vi "Stage Reference Follower.vi"(6 "stop":bool, 8 "Stage PID Cluster":T1={"Stage Z PID"={"Kp"=0.0005, "Kd"=0.001, "Ki"=0.0}, "Stage Y PID"={"Kp"=0.0003, "Kd"=0.01, "Ki"=0.0}, "Stage X PID"={"Kp"=0.0003, "Kd"=0.01, "Ki"=0.0}}, 9 "Stage cmd Posit [mm]":dbl[](array[numeric])=[6.0, 6.0, 6.0], 10 "error in":errorcluster, 11 "FPGA VI Reference In":refnum<k20>) -> (1 "Stage out Posit [mm]":dbl[](array[numeric])=[12.0, 0.0, 0.0], 2 "error out":errorcluster, 3 "FPGA VI Reference Out":refnum<k20>)   [LabVIEW 2016]
uses:
  <vilib>/Utility/error.llb/Error Cluster From Error Code.vi
  <vilib>/rvi/errors/niLvFpgaAdjustHostInterfaceError.vi
  <vilib>/rvi/interface/nirviReadWriteControl/nirviReadWriteControl.xnode
  FPGA Bitfiles/IRISSTrack_FPGATarget2_IRISSFPGAIORIO_4NTO9ubhv-c.lvbitx
  IRISS_FPGA_IO_RIO.vi
  Library/jmslib.lvlib
  NiFpgaLv.dll
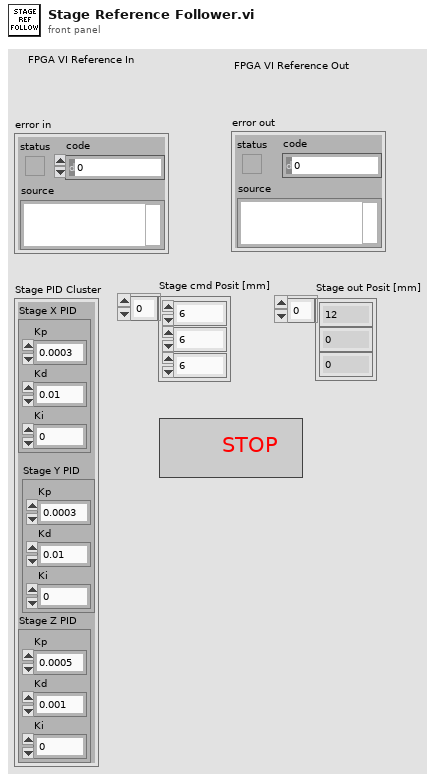
[diagram p1: front panel]
types:
  T1 = cluster{"Stage Z PID":cluster{"Kp":dbl, "Kd":dbl, "Ki":dbl}, "Stage Y PID":cluster{"Kp":dbl, "Kd":dbl, "Ki":dbl}, "Stage X PID":cluster{"Kp":dbl, "Kd":dbl, "Ki":dbl}}
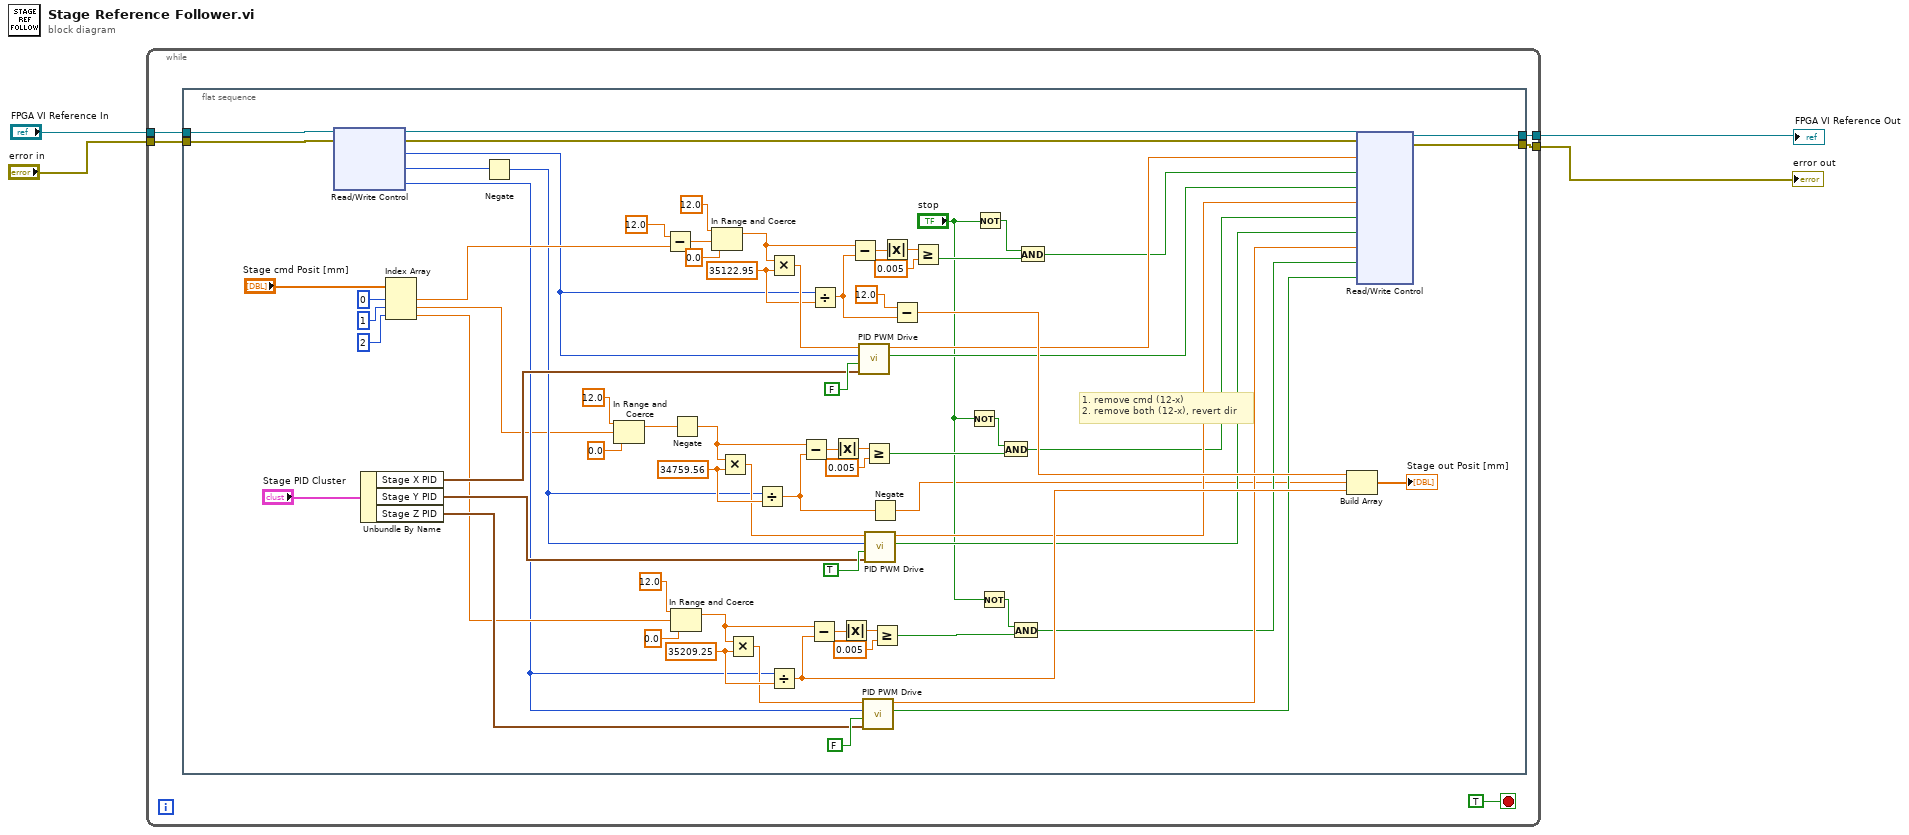
[diagram p0: block diagram]
diagram:
  n1 = while {
    tunnel: "FPGA VI Reference In" -> [w9]
    tunnel: "error in" -> [w8]
    tunnel: [w7] -> w1
    tunnel: [w6] -> w4
    stop <- TRUE stop-if-true
    n2 = flat-sequence {
      tunnel: w9 -> [w83]
      tunnel: w8 -> [w82]
      tunnel: [w22] -> w7
      tunnel: [w21] -> w6
      frame #0 {
        w49 = 35209.25 ("y")
        w63 = 34759.56 ("y")
        w78 = 35122.95 ("y")
        # "1. remove cmd (12-x)\n2. remove both (12-x), revert dir"
        n3 = xnode "Read/Write Control"("FPGA VI Reference In"=w83, "error in"=w82) -> ("FPGA VI Reference Out"=w24:refnum<k20>, "error out"=w23:errorcluster, "Position X"=w31:i32, "Position Y"=w16:i32, "Position Z"=w20:i32)
        n4 = Unbundle By Name("Stage PID Cluster") -> ("Stage X PID"=w56:cluster{"Kp":dbl, "Kd":dbl, "Ki":dbl}, "Stage Y PID"=w55:cluster{"Kp":dbl, "Kd":dbl, "Ki":dbl}, "Stage Z PID"=w43:cluster{"Kp":dbl, "Kd":dbl, "Ki":dbl})
        n5 = Index Array(array="Stage cmd Posit [mm]", index #1=0 ("index"), index #2=1 ("index"), index #3=2 ("index")) -> (element #1=w68:dbl, element #2=w10:dbl, element #3=w39:dbl)
        n6 = Negate(x=w16) -> (-x=w15:i32)
        n7 = In Range and Coerce(upper limit=12.0, x=w10, lower limit=0.0) -> (coerced(x)=w12:dbl)  [unwired: 1 out]
        n8 = Subtract(x=12.0 ("upper limit"), y=w68) -> (x-y=w72:dbl)
        n9 = In Range and Coerce(upper limit=12.0, x=w39, lower limit=0.0) -> (coerced(x)=w51:dbl)  [unwired: 1 out]
        n10 = Negate(x=w12) -> (-x=w11:dbl)
        n11 = In Range and Coerce(upper limit=12.0, x=w72, lower limit=0.0) -> (coerced(x)=w76:dbl)  [unwired: 1 out]
        n12 = Multiply(x=w11, y=w63) -> (x*y=w61:dbl)
        n13 = Multiply(x=w51, y=w49) -> (x*y=w47:dbl)
        n14 = Divide(x=w15, y=w63) -> (x/y=w13:dbl)
        n15 = Multiply(x=w76, y=w78) -> (x*y=w80:dbl)
        n16 = Divide(x=w20, y=w49) -> (x/y=w35:dbl)
        n17 = Subtract(x=w11, y=w13) -> (x-y=w65:dbl)
        n18 = Subtract(x=w51, y=w35) -> (x-y=w52:dbl)
        n19 = Divide(x=w31, y=w78) -> (x/y=w70:dbl)
        n20 = Absolute Value(x=w65) -> (abs(x)=w66:dbl)
        n21 = Absolute Value(x=w52) -> (abs(x)=w53:dbl)
        n22 = Subtract(x=w76, y=w70) -> (x-y=w75:dbl)
        n23 = call "PID PWM Drive.vi"("PID Gains"=w56, "Reverse Motor?"=FALSE, "Encoder Position"=w31, "Reference"=w80) -> ("Direction"=w30:bool, "Duty Cycle"=w33:dbl)  [unwired: 5 in, 1 out]
        n24 = call "PID PWM Drive.vi"("PID Gains"=w43, "Reverse Motor?"=FALSE, "Encoder Position"=w20, "Reference"=w47) -> ("Direction"=w25:bool, "Duty Cycle"=w27:dbl)  [unwired: 5 in, 1 out]
        n25 = Greater Or Equal?(x=w66, y=0.005) -> (x >= y?=w59:bool)
        n26 = call "PID PWM Drive.vi"("PID Gains"=w55, "Reverse Motor?"=TRUE, "Encoder Position"=w15, "Reference"=w61) -> ("Direction"=w28:bool, "Duty Cycle"=w32:dbl)  [unwired: 5 in, 1 out]
        n27 = Negate(x=w13) -> (-x=w14:dbl)
        n28 = Greater Or Equal?(x=w53, y=0.005) -> (x >= y?=w45:bool)
        n29 = Absolute Value(x=w75) -> (abs(x)=w74:dbl)
        n30 = Subtract(x=12.0 ("upper limit"), y=w70) -> (x-y=w36:dbl)
        n31 = Greater Or Equal?(x=w74, y=0.005) -> (x >= y?=w38:bool)
        n32 = Not(x="stop") -> (.not. x?=w58:bool)
        n33 = Not(x="stop") -> (.not. x?=w37:bool)
        n34 = Not(x="stop") -> (.not. x?=w44:bool)
        n35 = And(x=w58, y=w59) -> (x .and. y?=w29:bool)
        n36 = And(x=w44, y=w45) -> (x .and. y?=w26:bool)
        n37 = And(x=w37, y=w38) -> (x .and. y?=w19:bool)
        n38 = Build Array(w36, w14, w35) -> (→"Stage out Posit [mm]":dbl[])
        n39 = xnode "Read/Write Control"("FPGA VI Reference In"=w24, "error in"=w23, "X DC"=w33, "INHB X"=w19, "DIR X"=w30, "Y DC"=w32, "INHB Y"=w29, "DIR Y"=w28, "Z DC"=w27, "INHB Z"=w26, "DIR Z"=w25) -> ("FPGA VI Reference Out"=w22:refnum<k20>, "error out"=w21:errorcluster)
      }
    }
  }
  "error out" <- w4
  "FPGA VI Reference Out" <- w1
